vi "NewTemplate.GetBroadcasts.vi"(11 "NewTemplate in":refnum<class "CRON.lvclass">) -> (2 "TemplateModule":cluster{"Broadcasts":T1, "Broadcasts":T2}, 3 "NewTemplate out":refnum<class "CRON.lvclass">)   [LabVIEW 2024, in "CRON.lvclass"]
uses:
  CRON.lvclass
  RQMHCore/ModuleCore/StandardBroadcasts.ctl
  RQMHCore/Shared/Died.ctl
  RQMHCore/ModuleCore/Started.ctl
  Broadcast Events--cluster.ctl
  Stopped.ctl
  RQMHCore/ModuleCore/RQMHModule.lvclass/RQMHModule.ctl
  CRON.lvclass/CRON.ctl
  RQMHCore/ModuleCore/RQMHModule.lvclass
  C:/DevOps/CORTEX/JQMH/RQMHCore/ModuleCore/RQMHModule.lvclass
  C:/DevOps/CORTEX/JQMH/ModuleTemplates/CRON/CRON.lvclass
  RQMHCore/Shared/RQMHShared.lvlib
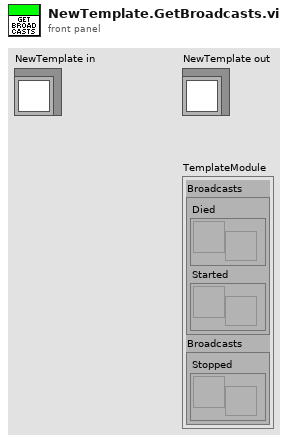
[diagram p1: front panel]
types:
  T1 = typedef "RQMHModule.lvclass/StandardBroadcasts.ctl" = cluster{"Died":refnum<user-event>, "Started":refnum<user-event>}
  T2 = typedef "CRON.lvclass/Broadcast Events--cluster.ctl" = cluster{"Stopped":refnum<user-event>}
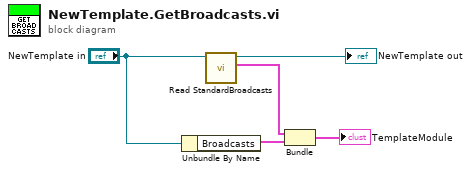
[diagram p0: block diagram]
diagram:
  n1 = Unbundle By Name("NewTemplate in") -> ("Broadcasts"=w5:T2)
  n2 = call "Read StandardBroadcasts.vi"("JQMHCore in"="NewTemplate in") -> ("Broadcasts"=w4:T1, "JQMHCore out"=→"NewTemplate out":refnum<class "CRON.lvclass">)  [unwired: 8 in, 1 out]
  n3 = Bundle("Broadcasts"=w4, "Broadcasts"=w5) -> (→"TemplateModule":cluster{"Broadcasts":T1, "Broadcasts":T2})  [unwired: 1 in]
